vi "Create Output File.vi"(6 "Local Data":T1, 8 "error in":errorcluster) -> (0 "error out":errorcluster, 4 "Local Data Out":T1)   [LabVIEW 2025]
uses:
  Controls/Local Data_Recording.ctl
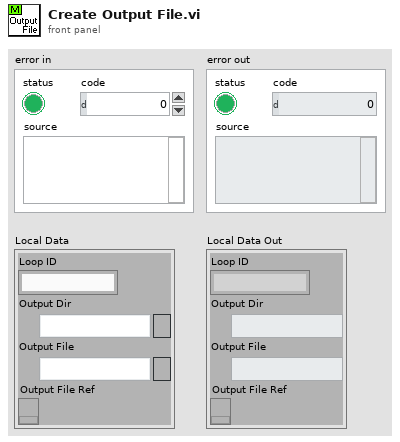
[diagram p1: front panel]
types:
  T1 = typedef "Local Data_Recording.ctl" = cluster{"Loop ID":string, "Output Dir":path, "Output File":path, "Output File Ref":refnum<k34>}
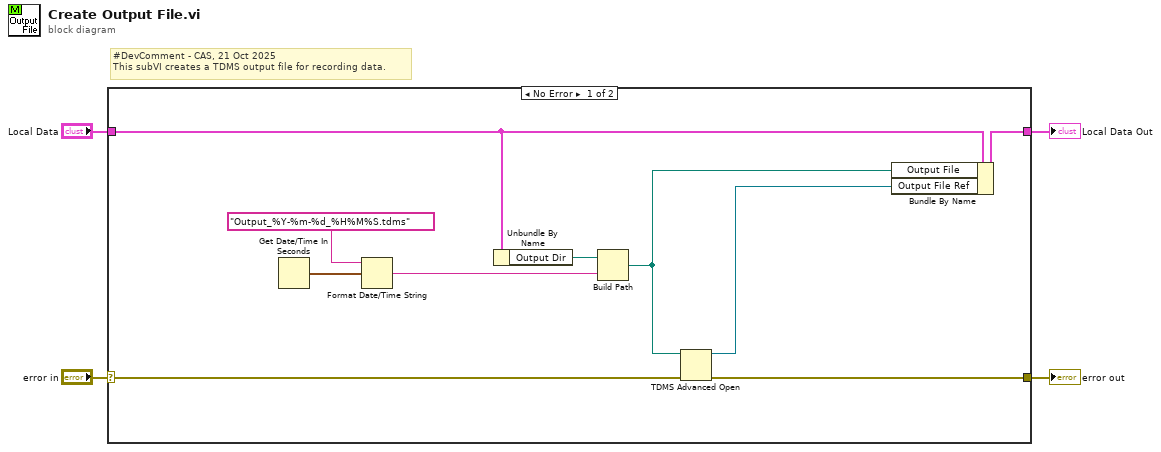
[diagram p0: block diagram]
diagram:
  # "#DevComment - CAS, 21 Oct 2025\nThis subVI creates a TDMS output file for recording data."
  n1 = case shown="No Error" "error in" {
    selector: "error in" -> [w10 w15]
    tunnel: "Local Data" -> [w13 w16]
    tunnel: [w9 w15] -> w2
    tunnel: [w14 w16] -> w1
    frame No Error {
      n2 = Get Date/Time In Seconds() -> (seconds since 1Jan1904=w12:timestamp)
      n3 = Format Date/Time String(time format string (%c)="Output_%Y-%m-%d_%H%M%S.tdms", seconds (now)=w12) -> (date/time string=w7:string)  [unwired: 1 in]
      n4 = Unbundle By Name(w13) -> ("Output Dir"=w8:path)
      n5 = Build Path(base path=w8, name or relative path=w7) -> (appended path=w5:path)
      n6 = TDMS Advanced Open(8:w10, 11:w5) -> (0:w9:errorcluster, 3:w6:refnum<k34>)  [unwired: 3 in, 1 out]
      n7 = Bundle By Name(cluster=w13, "Output File"=w5, "Output File Ref"=w6) -> (w14:T1)
    }
    frame Error {
    }
  }
  "error out" <- w2
  "Local Data Out" <- w1
